vi "testDBL2a.vi"() -> ()   [LabVIEW 2026]
panel:
  out "Waveform Graph":dbl[](graph)
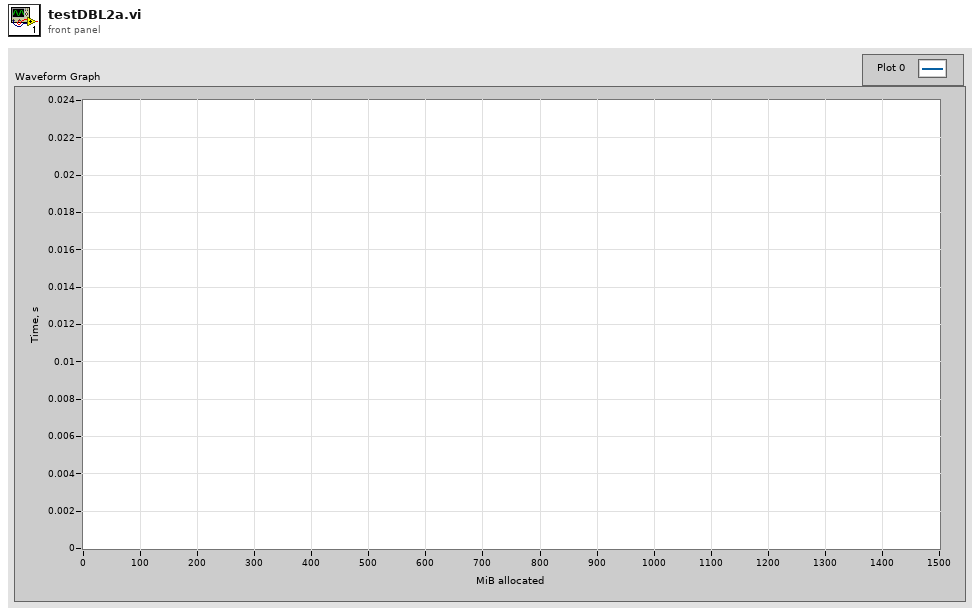
[diagram p1: front panel]
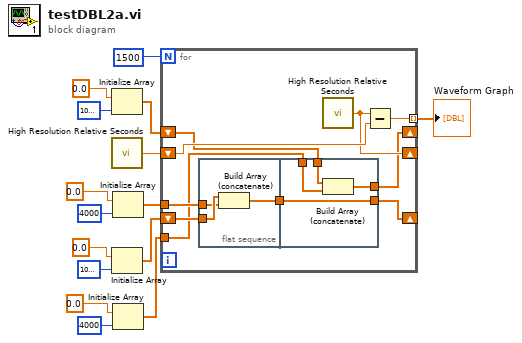
[diagram p0: block diagram]
diagram:
  n1 = Initialize Array(0.0 ("element"), 1048576 ("dimension size")) -> (w3:dbl[])
  n2 = call <vilib>:"High Resolution Relative Seconds.vi"() -> ("relative seconds"=w11:dbl)
  n3 = Initialize Array(0.0 ("element"), 1048576 ("dimension size")) -> (w13:dbl[])
  n4 = Initialize Array(0.0 ("element"), 4000 ("dimension size")) -> (w7:dbl[])
  n5 = Initialize Array(0.0 ("element"), 4000 ("dimension size")) -> (w6:dbl[])
  n6 = for {
    N: 1500 -> [_]
    shift-right: [w24] -> _
    shift-left: w13 -> [w25]
    shift-right: [w21] -> _
    shift-left: w11 -> [w23]
    tunnel: [w22] -> w10 mode=indexing
    tunnel: w7 -> [w20]
    shift-right: [w16] -> _
    shift-left: w3 -> [w18]
    tunnel: w6 -> [w17]
    n7 = flat-sequence {
      tunnel: w25 -> [w28]
      tunnel: w20 -> [w26]
      tunnel: [w27] -> w19
      tunnel: [w32] -> w24
      tunnel: w19 -> [w32]
      tunnel: w18 -> [w31]
      tunnel: w17 -> [w30]
      tunnel: [w29] -> w16
      frame #0 {
        n8 = Build Array (concatenate)(w28, w26) -> (w27:dbl[])
      }
      frame #1 {
        n9 = Build Array (concatenate)(w31, w30) -> (w29:dbl[])
      }
    }
    n10 = call <vilib>:"High Resolution Relative Seconds.vi"() -> ("relative seconds"=w21:dbl)
    n11 = Subtract(x=w21, y=w23) -> (x-y=w22:dbl)
  }
  "Waveform Graph" <- w10
